vi "Encoder to RPM.vi"(0 "CounterDevRef in":T1, 3 "error in (no error)":errorcluster, 4 "Ticks per Revolution":dbl) -> (7 "CounterDevRef out":T1, 8 "RPM":dbl, 9 "Stopped?":bool, 10 "error out":errorcluster)   [LabVIEW 2011]
uses:
  <vilib>/Rock Robotics/WPI/Counter/WPI_CounterDevRef.ctl
  <vilib>/Rock Robotics/SystemInterfaces/Counter/FPGA_CounterCtrSystemIndex.ctl
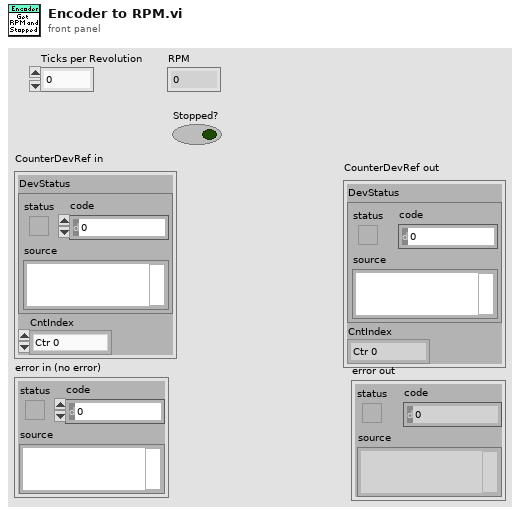
[diagram p1: front panel]
types:
  T1 = typedef "WPI_CounterDevRef.ctl" = cluster{"DevStatus":errorcluster, "CntIndex":T2}
  T2 = typedef "FPGA_CounterCtrSystemIndex.ctl" = enum8{"Ctr 0", "Ctr 1", "Ctr 2", "Ctr 3", "Ctr 4", "Ctr 5", "Ctr 6", "Ctr 7", "Invalid"}
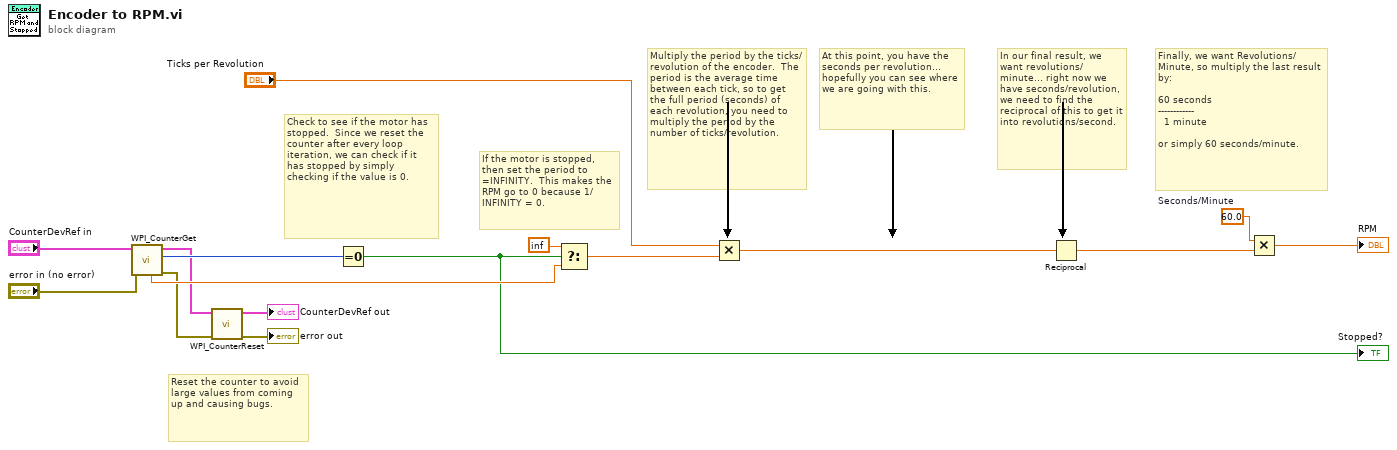
[diagram p0: block diagram]
diagram:
  w16 = 60.0  # Seconds/Minute
  # "Reset the counter to avoid large values from coming up and causing bugs."
  # "Finally, we want Revolutions/Minute, so multiply the last result by:\n\n60 seconds\n------------\n  1 minute\n\nor simply 60 seconds/minute."
  # "In our final result, we want revolutions/minute... right now we have seconds/revolution, we need to find the reciprocal of this to get it into revolutions/second."
  # "At this point, you have the seconds per revolution... hopefully you can see where we are going with this."
  # "Multiply the period by the ticks/revolution of the encoder.  The period is the average time between each tick, so to get the full period (seconds) of each revolution, you need to multiply the period by the number of ticks/revolution."
  # "If the motor is stopped, then set the period to =INFINITY.  This makes the RPM go to 0 because 1/INFINITY = 0."
  # "Check to see if the motor has stopped.  Since we reset the counter after every loop iteration, we can check if it has stopped by simply checking if the value is 0."
  n1 = call <vilib>:"WPI_CounterGet.vi"("error in (no error)"="error in (no error)", "CounterDevRef in"="CounterDevRef in") -> ("error out"=w3:errorcluster, "Value"=w6:i32, "CounterDevRef out"=w4:T1, "Period (sec)"=w9:dbl)  [unwired: 4 in, 2 out]
  n2 = call <vilib>:"WPI_CounterReset.vi"("error in (no error)"=w3, "CounterDevRef in"=w4) -> ("error out"=→"error out":errorcluster, "CounterDevRef out"=→"CounterDevRef out":T1)  [unwired: 8 in]
  n3 = Equal To 0?(x=w6) -> (x = 0?=w5:bool)
  "Stopped?" <- w5
  n4 = Select(t=inf, s=w5, f=w9) -> (s? t:f=w11:dbl)
  n5 = Multiply(x="Ticks per Revolution", y=w11) -> (x*y=w15:dbl)
  n6 = Reciprocal(x=w15) -> (1/x=w10:dbl)
  n7 = Multiply(x=w16, y=w10) -> (x*y=→"RPM":dbl)
